vi "Write PAS Coefficients.vi"(0 "Session Handle in":T1, 5 "Starting Address":u16=171 format="%x", 7 "Coefficients":dbl[](array[numeric]) format="%#_13g", 11 "error in (no error)":errorcluster) -> (4 "Session Handle out":T1, 15 "error out":errorcluster)   [LabVIEW 2015, in "PAS.lvclass"]
uses:
  PAS.lvclass
  Typedefs/Session Handle.ctl
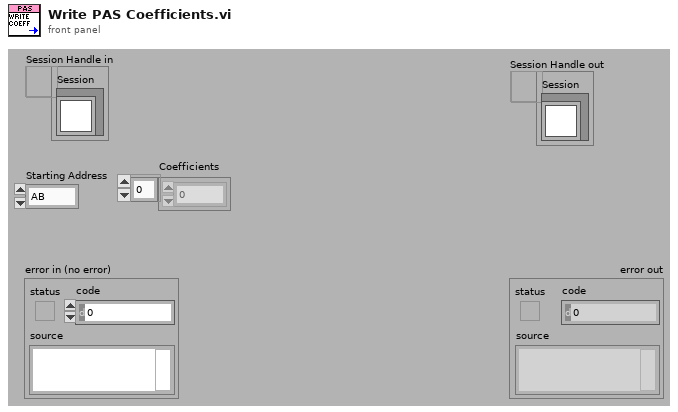
[diagram p1: front panel]
types:
  T1 = typedef "PAS.lvclass/Session Handle.ctl" = refnum<data-value>
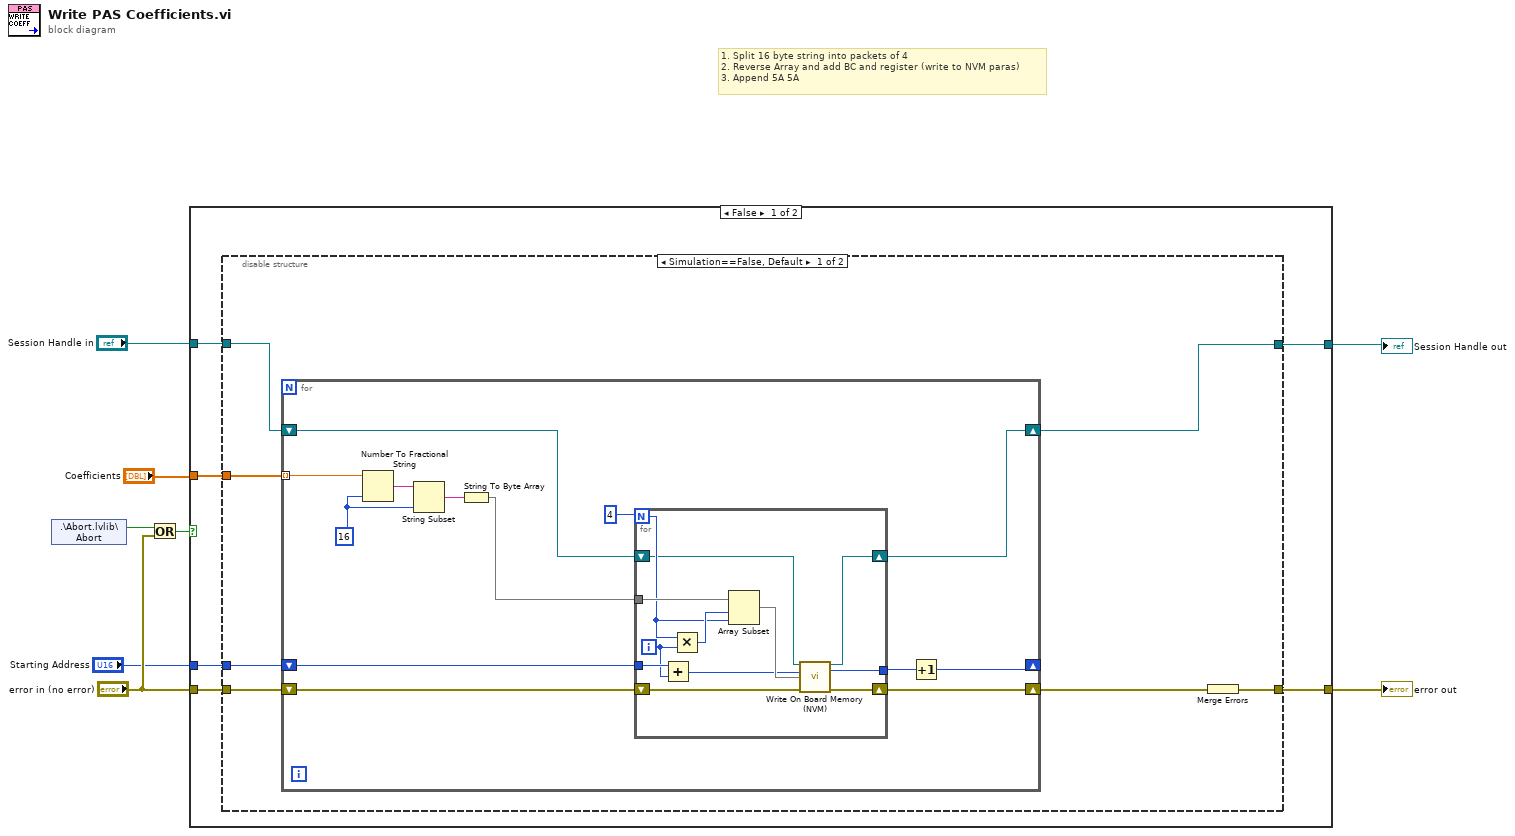
[diagram p0: block diagram]
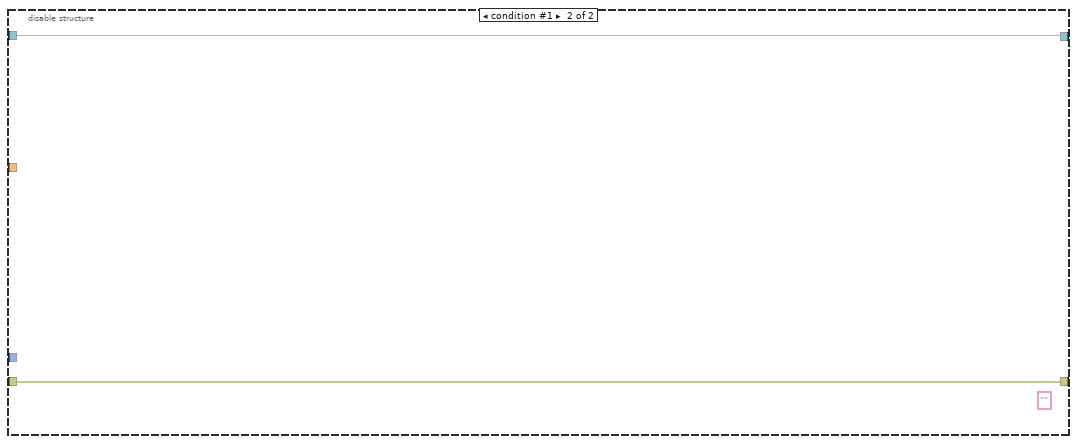
[diagram p2: hidden frame]
diagram:
  # "1. Split 16 byte string into packets of 4\n2. Reverse Array and add BC and register (write to NVM paras)\n3. Append 5A 5A"
  n1 = shared-variable ".\\Abort.lvlib\\Abort"() -> (w5:bool)  [unwired: 1 in, 1 out]
  n2 = Or(x=w5, y="error in (no error)") -> (x .or. y?=w3:bool)
  n3 = case shown="False" w3 {
    tunnel: [w14 w49] -> w7
    tunnel: [w13 w48] -> w6
    tunnel: "Session Handle in" -> [w12 w49]
    tunnel: "error in (no error)" -> [w11 w48]
    tunnel: "Starting Address" -> [w10 _]
    tunnel: "Coefficients" -> [w9 _]
    frame False {
      n4 = disable-structure shown="Simulation==False, Default" {
        disable-tunnel: [w15 w47] -> w14
        disable-tunnel: [w21 w46] -> w13
        disable-tunnel: w12 -> [w17 w47]
        disable-tunnel: w11 -> [w19 w46]
        disable-tunnel: w10 -> [w18 _]
        disable-tunnel: w9 -> [w20 _]
        frame condition #0 (active) {
          n5 = for {
            tunnel: w20 -> [w34] mode=indexing
            shift-right: [w25] -> w16
            shift-left: w19 -> [w30]
            shift-right: [w24] -> w15
            shift-left: w17 -> [w26]
            shift-right: [w22] -> _
            shift-left: w18 -> [w27]
            w32 = i16 16 ("precision (6)")
            n6 = Number To Fractional String(number=w34, precision (6)=w32) -> (F-format string=w33:string)  [unwired: 2 in]
            n7 = String Subset(string=w33, length (rest)=w32) -> (substring=w31:string)  [unwired: 1 in]
            n8 = String To Byte Array(string=w31) -> (unsigned byte array=w28:u8[])
            n9 = for {
              N: 4 -> [w42]
              tunnel: w28 -> [w44]
              shift-right: [w40] -> w25
              shift-left: w30 -> [w45]
              shift-right: [w38] -> w24
              shift-left: w26 -> [w39]
              tunnel: w27 -> [w37]
              tunnel: [w35] -> w23
              i -> [w36]
              n10 = Add(x=w37, y=w36) -> (x+y=w35:i32)
              n11 = Multiply(x=w42, y=w36) -> (x*y=w43:i32)
              n12 = Array Subset(array=w44, index=w43, length=w42) -> (w41:u8[])
              n13 = call "Write On Board Memory (NVM).vi"("Session Handle in"=w39, "Address"=w35, "Bytes to Write"=w41, "error in (no error)"=w45) -> ("Session Handle out"=w38:T1, "error out"=w40:errorcluster)  [unwired: 10 in]
            }
            n14 = Increment(x=w23) -> (x+1=w22:i32)
          }
          n15 = Merge Errors(w16) -> (w21:errorcluster)
        }
        frame condition #1 {
          (unwired) "" ("string")
        }
      }
    }
    frame True {
    }
  }
  "Session Handle out" <- w7
  "error out" <- w6
